vi "Get Parts.vi"(11 "Part list":string) -> (3 "Parts":map{string, i64}[](array[numeric]))   [LabVIEW 2021]
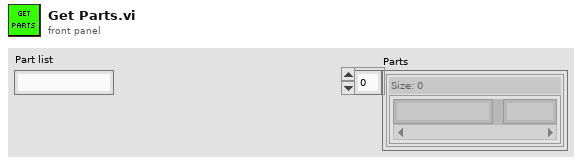
[diagram p1: front panel]
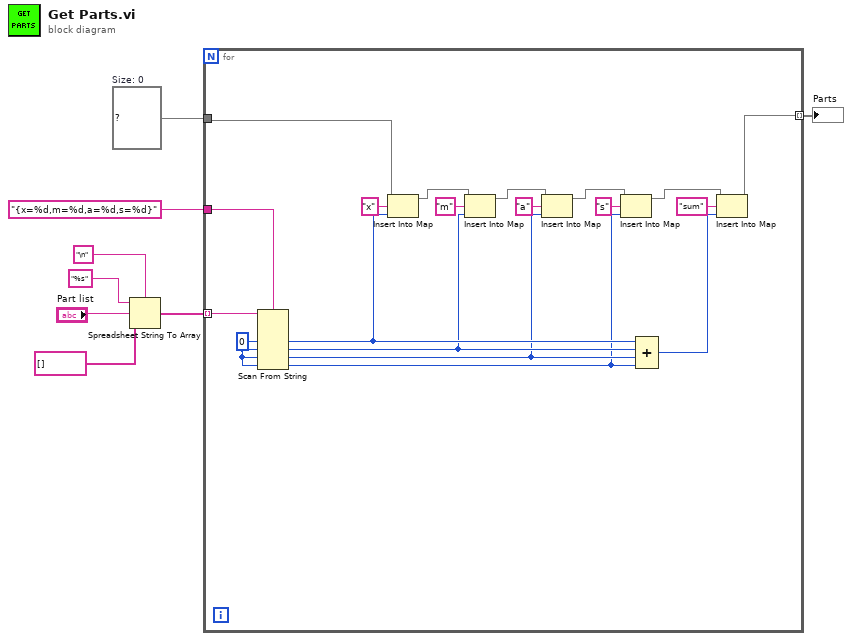
[diagram p0: block diagram]
diagram:
  w2 = map{string, i64} {}  # Size: 0
  n1 = Spreadsheet String To Array(delimiter (Tab)="\n", format string="%s", spreadsheet string="Part list", array type (2D Dbl)=string[] []) -> (array=w4:string[])
  n2 = for {
    tunnel: w4 -> [w27] mode=indexing
    tunnel: "{x=%d,m=%d,a=%d,s=%d}" -> [w26]
    tunnel: w2 -> [w24]
    tunnel: [w14] -> w1 mode=indexing
    w25 = i64 0 ("default value 1")
    n3 = Scan From String(format string=w26, input string=w27, default 1=w25, default 2=w25, default 3=w25, default 4=w25) -> (output 1=w13:i64, output 2=w12:i64, output 3=w11:i64, output 4=w10:i64)  [unwired: 2 in, 3 out]
    n4 = Insert Into Map(map in=w24, key="x", value=w13) -> (map out=w18:map{string, i64})  [unwired: 2 out]
    n5 = Insert Into Map(map in=w18, key="m", value=w12) -> (map out=w17:map{string, i64})  [unwired: 2 out]
    n6 = Insert Into Map(map in=w17, key="a", value=w11) -> (map out=w16:map{string, i64})  [unwired: 2 out]
    n7 = Insert Into Map(map in=w16, key="s", value=w10) -> (map out=w15:map{string, i64})  [unwired: 2 out]
    n8 = Compound Arithmetic op=ADD(w13, w12, w11, w10) -> (w9:i64)
    n9 = Insert Into Map(map in=w15, key="sum", value=w9) -> (map out=w14:map{string, i64})  [unwired: 2 out]
  }
  "Parts" <- w1
